vi "Setup Menu Bar.vi"(8 "error in (no error)":errorcluster, 11 "menu reference":refnum<k9>) -> (0 "error out":errorcluster)   [LabVIEW 2017, in "Message Log.lvclass"]
uses:
  Message Log.lvclass
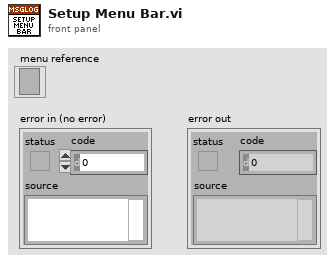
[diagram p1: front panel]
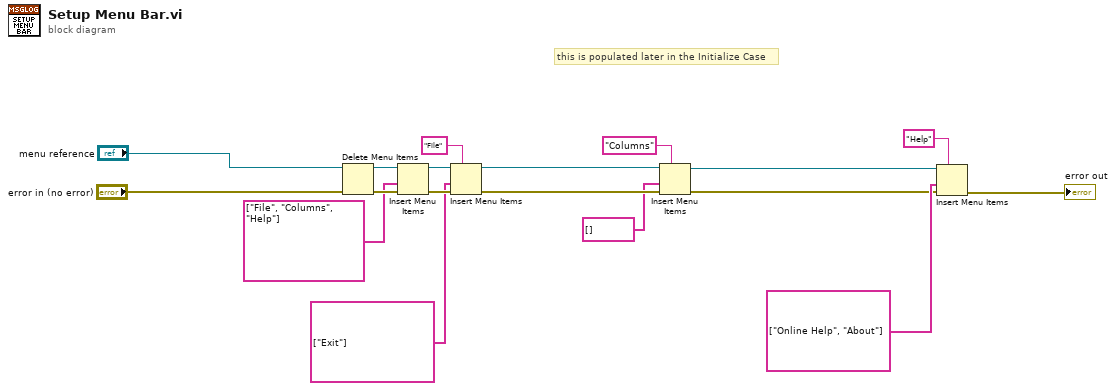
[diagram p0: block diagram]
diagram:
  # "this is populated later in the Initialize Case"
  n1 = Delete Menu Items(6:"error in (no error)", 9:"menu reference") -> (0:w18:errorcluster, 3:w17:refnum<k9>)  [unwired: 2 in]
  n2 = Insert Menu Items(6:w18, 7:string[] ["File", "Columns", "Help"] ("L10n_item tags 1"), 9:w17) -> (0:w14:errorcluster, 3:w13:refnum<k9>)  [unwired: 3 in, 1 out]
  n3 = Insert Menu Items(5:"File" ("L10n_menu tag"), 6:w14, 7:string[] ["Exit"] ("L10n_item tags 2"), 9:w13) -> (0:w5:errorcluster, 3:w2:refnum<k9>)  [unwired: 2 in, 1 out]
  n4 = Insert Menu Items(5:"Columns" ("L10n_menu tag"), 6:w5, 7:string[] [] ("item tags"), 9:w2) -> (0:w4:errorcluster, 3:w3:refnum<k9>)  [unwired: 2 in, 1 out]
  n5 = Insert Menu Items(5:"Help" ("L10n_menu tag"), 6:w4, 7:string[] ["Online Help", "About"] ("L10n_item tags 2"), 9:w3) -> (0:→"error out":errorcluster)  [unwired: 2 in, 2 out]
